vi "push.vi"   [LabVIEW 2017]
uses:
  <vilib>/myRIO/Instrument Drivers/Onboard IO/DIO/typedefs/DIO Reference.ctl
  <vilib>/myRIO/Common/Instrument Driver Framework/Utilities/typedefs/myRIO Generic Hardware Reference.ctl
  <vilib>/myRIO/Common/Instrument Driver Framework/Utilities/typedefs/Hardware Version Enum.ctl
  <vilib>/myRIO/Common/Instrument Driver Framework/Utilities/typedefs/myRIO v1.0 Reference.ctl
  <vilib>/myRIO/Common/Instrument Driver Framework/Utilities/typedefs/Generic FPGA Reference.ctl
  <vilib>/myRIO/Common/Instrument Driver Framework/myRIO v1.0/DIO/typedefs/DIO Channels List.ctl
  <vilib>/myRIO/Common/Instrument Driver Framework/myRIO v1.0/DIO/typedefs/DIO Channels Enum.ctl
  <vilib>/userdefined/High Color/nirio_resource_hc.ctl
  <vilib>/myRIO/Common/Instrument Driver Framework/Utilities/vis/Is FPGA Ref Available.vi
  <vilib>/myRIO/Common/Instrument Driver Framework/myRIO v1.0/DIO/vis/myRIO v1.1 Open DIO.vi
  <vilib>/myRIO/Instrument Drivers/Onboard IO/DIO/vis/Read.vi
  <vilib>/myRIO/Common/Instrument Driver Framework/Utilities/vis/Validate Channels.vi
  <vilib>/myRIO/Common/Instrument Driver Framework/myRIO v1.0/DIO/vis/myRIO v1.0 Reserve DIO.vi
  <vilib>/myRIO/Common/Instrument Driver Framework/myRIO v1.0/Resource Manager/vis/myRIO v1.0 Reserve Channel List.vi
  <vilib>/myRIO/Common/Instrument Driver Framework/myRIO v1.0/DIO/vis/myRIO v1.0 Build MUX Configuration DIO.vi
  <vilib>/myRIO/Common/Instrument Driver Framework/myRIO v1.0/Resource Manager/vis/myRIO v1.0 Reserve Channel.vi
  <vilib>/myRIO/Common/Instrument Driver Framework/myRIO v1.0/Resource Manager/vis/myRIO v1.0 Unreserve Channel.vi
  <vilib>/myRIO/Common/Instrument Driver Framework/myRIO v1.0/Resource Manager/vis/myRIO v1.0 Create Configuration List.vi
  <vilib>/myRIO/Common/Instrument Driver Framework/myRIO v1.0/Resource Manager/vis/myRIO v1.0 Build Mutex Name.vi
  <vilib>/Utility/VariantDataType/GetNumericInfo.vi
  <vilib>/Utility/error.llb/Error Cluster From Error Code.vi
  <vilib>/myRIO/Common/Instrument Driver Framework/myRIO v1.0/myRIO v1.1 Open.vi
  <vilib>/myRIO/Common/Instrument Driver Framework/Utilities/vis/IO Manager.vi
  <vilib>/myRIO/Common/Instrument Driver Framework/Utilities/vis/Configuration Manager.vi
  <vilib>/myRIO/Common/Instrument Driver Framework/myRIO v1.0/Resource Manager/vis/myRIO v1.0 Configure IO.vi
  <vilib>/myRIO/Common/Instrument Driver Framework/myRIO v1.0/myRIO v1.0 Close.vi
  <vilib>/myRIO/Common/Instrument Driver Framework/myRIO v1.0/DIO/vis/myRIO v1.0 Read DIO.vi
  <vilib>/myRIO/Express VI/Onboard IO/DI/DI Express VI.xnode
  <vilib>/myRIO/Instrument Drivers/Onboard IO/DIO/vis/myRIO DIO Open.xnode
  <vilib>/myRIO/Instrument Drivers/Onboard IO/DIO/DIO.lvlib
types:
  T1 = enum16{"hold", "f", "fl", "fr", "l", "r", "b", "bl", "br"}
  T2 = typedef "DIO.lvlib/DIO Reference.ctl" = cluster{"myRIO Reference":T3, "DIO Channels List":T7}
  T3 = typedef "myRIO Generic Hardware Reference.ctl" = cluster{"myRIO Model":T4, "myRIO Hardware Reference":T5}
  T4 = typedef "Hardware Version Enum.ctl" = enum16{"Unknown", "myRIO-1900", "myRIO-1950", "roboRIO", "NI ELVIS RIO CM"}
  T5 = typedef "myRIO v1.0 Reference.ctl" = cluster{"Generic FPGA Reference":T6, "Allow multiple opens":bool}
  T6 = typedef "Generic FPGA Reference.ctl" = refnum<k20>
  T7 = typedef "DIO Channels List.ctl" = T8[]
  T8 = typedef "DIO Channels Enum.ctl" = enum16{"Not Connected", "C/DIO0", "C/DIO1", "C/DIO2", "C/DIO3", "C/DIO4", "C/DIO5", "C/DIO6", "C/DIO7", "A/DIO0", "A/DIO1", "A/DIO2", "A/DIO3", "A/DIO4", "A/DIO5", "A/DIO6", "A/DIO7", "A/DIO8", "A/DIO9", "A/DIO10", "A/DIO11", "A/DIO12", "A/DIO13", "A/DIO14", "A/DIO15", "B/DIO0", "B/DIO1", "B/DIO2", "B/DIO3", "B/DIO4", "B/DIO5", "B/DIO6", "B/DIO7", "B/DIO8", "B/DIO9", "B/DIO10", "B/DIO11", "B/DIO12", "B/DIO13", "B/DIO14", "B/DIO15", "LED0", "LED1", "LED2", "LED3", "Button0", "DIO/DIO0", "DIO/DIO1", "DIO/DIO2", "DIO/DIO3", "DIO/DIO4", "DIO/DIO5", "DIO/DIO6", "DIO/DIO7", "DIO/DIO8", "DIO/DIO9", "SPI/CS0", "SPI/CS1", "SPI/CS2", "SPI/CS3", "LED RADIO (Green)", "LED RADIO (Red)", "LED COMM (Green)", "LED COMM (Red)", "LED MODE (Green)", "LED MODE (Red)"}
  T9 = typedef "nirio_resource_hc.ctl" = tag
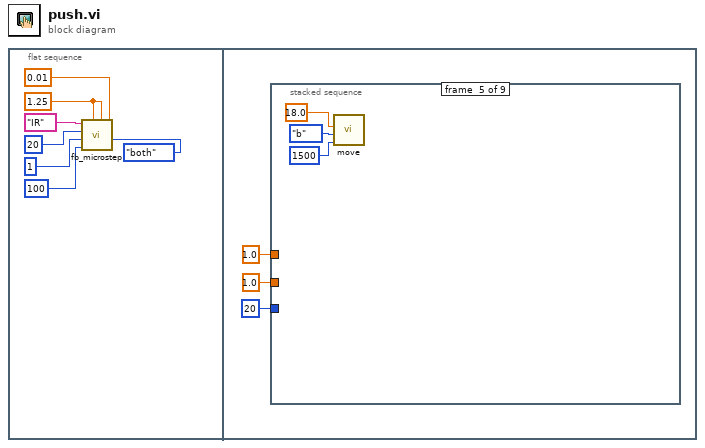
[diagram p0: block diagram]
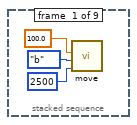
[diagram p2: hidden frame]
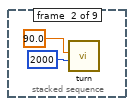
[diagram p3: hidden frame]
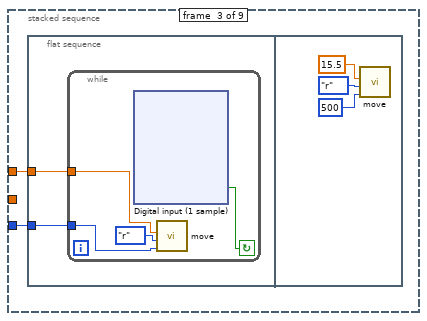
[diagram p4: hidden frame]
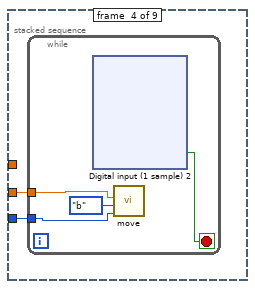
[diagram p5: hidden frame]
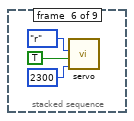
[diagram p6: hidden frame]
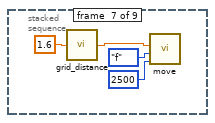
[diagram p7: hidden frame]
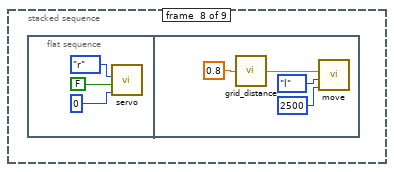
[diagram p8: hidden frame]
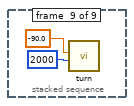
[diagram p9: hidden frame]
diagram:
  n1 = flat-sequence {
    frame #0 {
      w7 = 1.25 ("taget_IR_R")
      n2 = call "fb_microstep.vi"("Sensor"=enum16{"l", "r", "both"}."both", "precision"=0.01, "taget_IR_L"=w7, "taget_IR_R"=w7, "SamplingNUM"=100, "Step"=1, "Delay"=20, "Stop Mode"="IR") -> ()  [unwired: 3 in, 1 out]
    }
    frame #1 {
      n3 = stacked-sequence {
        tunnel: 1.0 ("D") -> [_ _ _ w64 _ _ _ _ _]
        tunnel: 1.0 ("D") -> [_ _ w17 _ _ _ _ _ _]
        tunnel: u32 20 ("delay") -> [_ _ w16 w63 _ _ _ _ _]
        frame #0 {
          n4 = call "move.vi"("delay"=u32 2500, "Enum"=T1."b", "D"=100.0) -> ()  [unwired: 9 in]
        }
        frame #1 {
          n5 = call "turn.vi"("delay"=u32 2000, "Carzeta"=90.0) -> ()  [unwired: 10 in]
        }
        frame #2 {
          n6 = flat-sequence {
            tunnel: w17 -> [w19]
            tunnel: w16 -> [w18]
            frame #0 {
              n7 = while {
                tunnel: w19 -> [w21]
                tunnel: w18 -> [w20]
                stop <- w22 continue-if-true
                n8 = xnode "Digital input (1 sample)"() -> ("R (A/DIO1 (Pin 13))"=w22:bool)  [unwired: 1 in, 2 out]
                n9 = call "move.vi"("delay"=w20, "Enum"=T1."r", "D"=w21) -> ()  [unwired: 9 in]
              }
            }
            frame #1 {
              n10 = call "move.vi"("delay"=u32 500, "Enum"=T1."r", "D"=15.5) -> ()  [unwired: 9 in]
            }
          }
        }
        frame #3 {
          n11 = while {
            tunnel: w64 -> [w66]
            tunnel: w63 -> [w65]
            stop <- w67 stop-if-true
            n12 = xnode "Digital input (1 sample) 2"() -> ("R (A/DIO1 (Pin 13))"=w67:bool)  [unwired: 1 in, 2 out]
            n13 = call "move.vi"("delay"=w65, "Enum"=T1."b", "D"=w66) -> ()  [unwired: 9 in]
          }
        }
        frame #4 {
          n14 = call "move.vi"("delay"=u32 1500, "Enum"=T1."b", "D"=18.0) -> ()  [unwired: 9 in]
        }
        frame #5 {
          n15 = call "servo.vi"("delay"=u32 2300, "in=true\nout = false"=TRUE ("in=true\nout = false"), "left-right"=enum16{"r", "l"}."r") -> ()  [unwired: 9 in]
        }
        frame #6 {
          n16 = call "grid_distance.vi"("x"=1.6) -> ("distance_mm"=w114:dbl)
          n17 = call "move.vi"("delay"=u32 2500, "Enum"=T1."f", "D"=w114) -> ()  [unwired: 9 in]
        }
        frame #7 {
          n18 = flat-sequence {
            frame #0 {
              n19 = call "servo.vi"("delay"=u32 0, "in=true\nout = false"=FALSE ("in=true\nout = false"), "left-right"=enum16{"r", "l"}."r") -> ()  [unwired: 9 in]
            }
            frame #1 {
              n20 = call "grid_distance.vi"("x"=0.8) -> ("distance_mm"=w121:dbl)
              n21 = call "move.vi"("delay"=u32 2500, "Enum"=T1."l", "D"=w121) -> ()  [unwired: 9 in]
            }
          }
        }
        frame #8 {
          n22 = call "turn.vi"("delay"=u32 2000, "Carzeta"=-90.0) -> ()  [unwired: 10 in]
        }
      }
    }
  }
